vi "Drive Roll Maneuver.vi"(7 "Reset?":bool, 8 "Backwards?":bool, 10 "Alt Side":bool) -> (1 "X":dbl, 2 "Y":dbl, 3 "Steer":dbl)   [LabVIEW 2013]
uses:
  <vilib>/Analysis/coordinate.llb/2D Cartesian Coordinate Rotation (Scalar).vi
  Robot Global Data.vi
  <vilib>/Rock Robotics/WPI/Gyro/WPI_GyroRefNum Registry Get.vi
  <vilib>/Rock Robotics/WPI/Gyro/WPI_GyroGetAngle.vi
  <vilib>/Analysis/NI_AALPro.lvlib
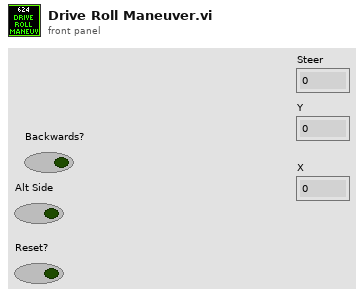
[diagram p1: front panel]
types:
  T1 = typedef "Dashboard UDP Packet.ctl" = cluster{"Camera":T2, "Gyro":T3, "Encoder":T5, "Auto Shift":T6, "Auton":T7, "Drive/Ramp X":dbl, "Drive/Ramp Y":dbl, "Drive/Battery Cutoff":dbl, "Pressure/Compressor Min Voltage":dbl, "Pressure/Compressor Delay":dbl, "Controller/Strafe Correction":bool, "Shooter":T8, "Rollers":T9, "Abort":bool, "Finish":bool, "IR Halo Sustain Time":dbl, "Disable Compressor":bool, "Center Omni Drive Delay":i32, "Vision Mode":T10, "Radius Throttle":bool, "Fieldcentric":T11, "Roll":T12, "Stick Deadband":dbl}
  T2 = typedef "Camera Controls.ctl" = cluster{"Camera/View Angle X":dbl, "Camera/Goal Track Timeout":dbl, "Camera/View Angle Y":dbl, "Camera/Goal Exposure":dbl, "Camera/Vision Receive Timeout":dbl, "Camera/Offset 1":dbl, "Camera/Offset 2":dbl}
  T3 = typedef "Gyro Controls.ctl" = cluster{"Gyro/Angle Tolerance":dbl, "Gyro/Steer Closeness Threshold":dbl, "Steer PID":T4, "Steer Close PID":T4}
  T4 = typedef "PID Params.ctl" = cluster{"max":dbl, "min":dbl, "P":dbl, "I":dbl, "D":dbl}
  T5 = typedef "Encoder Controls.ctl" = cluster{"Encoders/Reset":bool, "Encoders/Omni Constant":dbl, "Encoders/Omni Tick Constant":dbl, "Encoders/Left Constant":dbl, "Encoders/Right Constant":dbl, "Encoders/Right Tick Constant":dbl}
  T6 = typedef "Auto Shift Controls.ctl" = cluster{"AutoShift/Upshift Throttle Accel":dbl, "AutoShift/Speed Threshold":dbl, "AutoShift/Upshift Throttle":dbl, "AutoShift/Upshift Accel":dbl, "AutoShift/Downshift Accel":dbl, "AutoShift/Downshift Throttle":dbl, "AutoShift/Delay":dbl, "AutoShift/Enabled":bool}
  T7 = typedef "Auton Controls.ctl" = cluster{"Auton/Left Shoot X-Coord":dbl, "Auton/Right Shoot X-Coord":dbl, "DistDrive/Distance Stop Threshold":dbl, "DistDrive/Max Stop Speed":dbl, "Auton/Back Piston Time":dbl, "Auton/Manual Hot":bool, "Auton/Manual Hot Right":bool, "Default X PID":T4, "Default Y PID":T4}
  T8 = typedef "Shooter Controls.ctl" = cluster{"Shooter/Reset Time":dbl, "Shooter/Release Delay":dbl, "Shooter/Pressure Steady Time":dbl, "Shooter/Misfire Delay":dbl, "Shooter/Ball Settle Time":dbl, "Shooter/Line IR Delay":dbl, "Pressure/Upper PSI Time":dbl, "Pressure/Lower PSI Time":dbl, "Shooter/Punch Delay":dbl, "Shooter/Target Pressure":dbl, "Pressure/Line B":dbl, "Pressure/Line M":dbl, "Pressure/Shooter M":dbl, "Pressure/Shooter B":dbl, "Halo Time":dbl, "Soft Release Delay":dbl, "Soft Unpin Delay":dbl, "Soft Shoot Delay":dbl}
  T9 = typedef "Roller Controls.ctl" = cluster{"Roller/Load IRs Verify Time":dbl, "Roller/Center IR Latch Time":dbl, "Roller/Speed Front":dbl, "Roller/Speed Back":dbl, "Roller/Entry Timeout":dbl, "Roller/To Center Timeout":dbl, "Roller/Sustain Time":dbl, "Roller/Verify Center Time":dbl}
  T10 = typedef "Vision Mode.ctl" = enum16{"Normal", "Extreme Left", "Extreme Right"}
  T11 = typedef "Fieldcentric Controls.ctl" = cluster{"Relative Angle":bool, "Point Robot":bool, "X/Y ratio low":dbl, "Steering Gain":dbl, "Force Omni Down":bool, "Enable":bool, "X/Y ratio high":dbl}
  T12 = typedef "Roll Maneuver.ctl" = cluster{"X 1":dbl, "Y 1":dbl, "Y 2":dbl, "X 2":dbl, "Y 3":dbl, "X 3":dbl, "Time 1":i32, "Time 2":i32, "Time 3":i32, "Angle Start":dbl, "Angle End":dbl, "Angle Linearity":dbl}
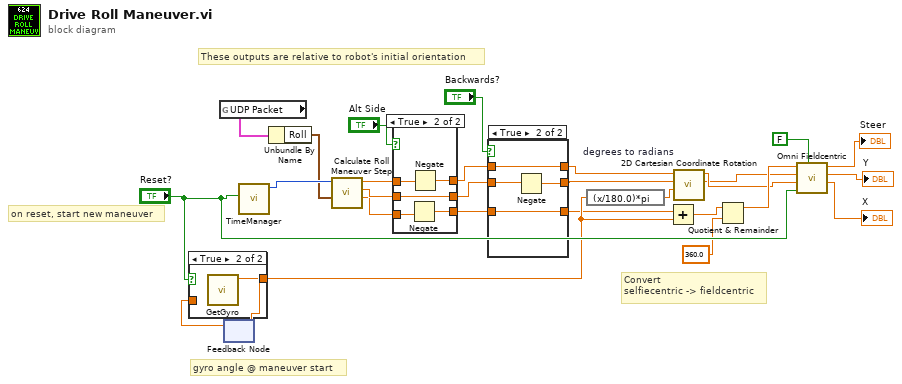
[diagram p0: block diagram]
diagram:
  # "Convert \nselfiecentric -> fieldcentric"
  # "gyro angle @ maneuver start"
  # "These outputs are relative to robot's initial orientation"
  # "on reset, start new maneuver"
  n1 = global read "Robot Global Data.vi" "UDP Packet"() -> (w26:T1)
  n2 = feedback #1() -> (w19:dbl)  [unwired: 1 in]
  n3 = case shown="True" "Reset?" {
    tunnel: [w28 w29] -> w8
    tunnel: w19 -> [w28 _]
    frame False {
    }
    frame True {
      n4 = call "GetGyro.vi"() -> ("Angle"=w29:dbl)  [unwired: 9 in, 2 out]
    }
  }
  n5 = feedback-in #1(w8) -> ()
  n6 = call "TimeManager.vi"("Reset?"="Reset?") -> ("Time Since Reset"=w27:u32)  [unwired: 9 in, 1 out]
  n7 = Unbundle By Name(w26) -> ("Roll"=w25:T12)
  n8 = call "Calculate Roll Maneuver Step.vi"("Roll"=w25, "Time"=w27) -> ("Angle"=w12:dbl, "Y"=w13:dbl, "X"=w14:dbl)  [unwired: 6 in, 1 out]
  n9 = case shown="True" "Alt Side" {
    tunnel: w14 -> [w32 w37]
    tunnel: [w32 w36] -> w7
    tunnel: w13 -> [w31 w35]
    tunnel: [w31 w35] -> w4
    tunnel: w12 -> [w30 w34]
    tunnel: [w30 w33] -> w2
    frame False {
    }
    frame True {
      n10 = Negate(x=w34) -> (-x=w33:dbl)
      n11 = Negate(x=w37) -> (-x=w36:dbl)
    }
  }
  n12 = case shown="True" "Backwards?" {
    tunnel: w7 -> [w40 w44]
    tunnel: [w40 w44] -> w6
    tunnel: w4 -> [w39 w42]
    tunnel: [w39 w41] -> w3
    tunnel: w2 -> [w38 w43]
    tunnel: [w38 w43] -> w1
    frame False {
    }
    frame True {
      n13 = Negate(x=w42) -> (-x=w41:dbl)
    }
  }
  n14 = expression code="(x/180.0)*pi" "degrees to radians"(w8) -> (w9:dbl)
  n15 = Add(x=w1, y=w8) -> (x+y=w18:dbl)
  n16 = call-poly <vilib>:"2D Cartesian Coordinate Rotation.vi"("theta"=w9, "y"=w3, "x"=w6) -> ("y out"=w10:dbl, "x out"=w11:dbl)  [unwired: 6 in, 1 out]
  n17 = Quotient & Remainder(x=w18, y=360.0) -> (x-y*floor(x/y)=w16:dbl)  [unwired: 1 out]
  n18 = call "Omni Fieldcentric.vi"("Point Robot"=FALSE, "reinit?"="Reset?", "axis 1 (x)"=w11, "axis 2 (y)"=w10, "Steer Target Angle"=w16) -> ("Translation X"=→"X":dbl, "Translation Y"=→"Y":dbl, "Rotation"=→"Steer":dbl)  [unwired: 4 in]
